vi "Create JUnit Root.vi"(8 "Error In (No Error)":errorcluster, 11 "Test Suites Atrributes":T1={"name"="", "tests"=-1, "failures"=-1, "errors"=-1, "time"=-1.0, "disabled"=-1, "skipped"=-1, "skips"=-1, "timestamp"=-1.0, "hostname"="", "id"="", "package"="", "assertions"=-1, "file"="", "skip"="", "log"="", "url"=""}) -> (0 "Error Out":errorcluster, 2 "Teststuites Ref":refnum<k20>, 3 "File Ref Out":refnum<k20>)   [LabVIEW 2013, in "JUnit API.lvlib"]
doc: "Creates a new XML file for JUnit reporting and instantiates the teststuites root node."
uses:
  JUnit API.lvlib
  Controls/Test Suite Attribute Values.ctl
  <vilib>/NI/Simple XML/_polymorphics/Create Tag - Root.vi
  <vilib>/xml/NI_XML.lvlib
  <vilib>/NI/Simple XML/Simple XML.lvlib
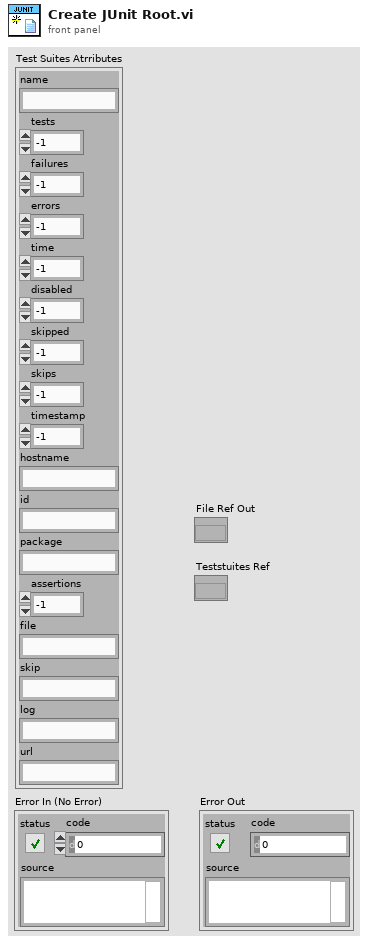
[diagram p1: front panel]
types:
  T1 = typedef "JUnit API.lvlib/Test Suite Attribute Values.ctl" = cluster{"name":string, "tests":i32, "failures":i32, "errors":i32, "time":dbl, "disabled":i32, "skipped":i32, "skips":i32, "timestamp":dbl, "hostname":string, "id":string, "package":string, "assertions":i32, "file":string, "skip":string, "log":string, "url":string}
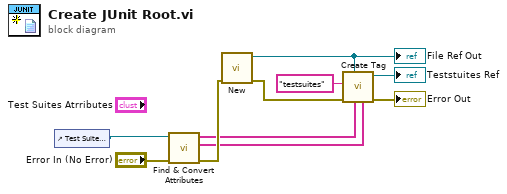
[diagram p0: block diagram]
diagram:
  n1 = control-ref of="Test Suites Atrributes"() -> (w1:refnum<vi>)
  n2 = call "Find & Convert Attributes.vi"("Error In"="Error In (No Error)", "Cluster in"=w1) -> ("Error Out"=w10:errorcluster, "Attribute Values"=w8:string[], "Attribute Names"=w9:string[])  [unwired: 7 in]
  n3 = call <vilib>:"New.vi"("error in (no error)"=w10) -> ("error out"=w3:errorcluster, "DOM document out"=w6:refnum<k20>)  [unwired: 7 in]
  "File Ref Out" <- w6
  n4 = call-poly <vilib>:"Create Tag.vi"("Attr Values"=w8, "Attr Names"=w9, "DOM document reference"=w6, "error in (no error)"=w3, "Tag Name"="testsuites") -> ("error out"=→"Error Out":errorcluster, "Element reference"=→"Teststuites Ref":refnum<k20>)  [unwired: 5 in]
